vi "PSA Alignment Progress Bar.vi"(8 "error in (no error)":errorcluster, 10 "Time Target (s)":dbl=65.0 format="%#_13g", 11 "VISA resource in":refnum<visa-resource-name>) -> (0 "error out":errorcluster, 2 "Complete?":bool, 3 "VISA resource out":refnum<visa-resource-name>)   [LabVIEW 2014]
panel:
  out "Elapsed Time to Alignment Completion":u32(slide) scale=0.0..60.0
  out "Elapsed Time (s)":u32 format="%<%H:%M:%S>t"
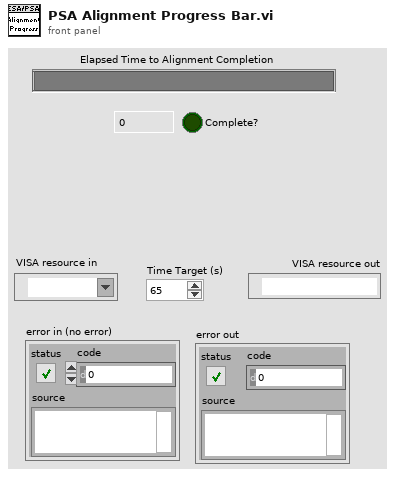
[diagram p1: front panel]
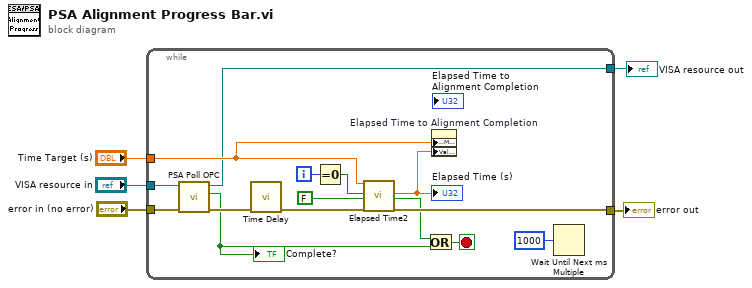
[diagram p0: block diagram]
diagram:
  n1 = while {
    tunnel: [w19] -> w2
    tunnel: "error in (no error)" -> [w12]
    tunnel: "VISA resource in" -> [w10]
    tunnel: "Time Target (s)" -> [w13]
    tunnel: [w6] -> w1
    i -> [w16]
    stop <- w17 stop-if-true
    n2 = call "PSA Poll OPC.vi"("error in (no error)"=w12, "VISA resource name"=w10) -> ("error out"=w11:errorcluster, "OPC Complete?"=w9:bool, "VISA resource name out"=w6:refnum<visa-resource-name>)  [unwired: 7 in]
    "Complete?" <- w9
    n3 = call "Time Delay"("error in (no error)"=w11) -> ("error out"=w20:errorcluster)  [unwired: 10 in]
    n4 = Equal To 0?(x=w16) -> (x = 0?=w15:bool)
    n5 = call "Elapsed Time2"("Time Target (s)"=w13, "Reset"=w15, "Auto Reset"=FALSE, "error in (no error)"=w20) -> ("Elapsed Time (s)"=w8:dbl, "Time has Elapsed"=w18:bool, "error out"=w19:errorcluster)  [unwired: 8 in, 5 out]
    "Elapsed Time (s)" <- w8
    n6 = Or(x=w18, y=w9) -> (x .or. y?=w17:bool)
    n7 = property on="Elapsed Time to Alignment Completion" class="Slide (strict)"("Scale.Maximum"=w13, "Value"=w8) -> ()  [unwired: 2 in, 2 out]
    n8 = Wait Until Next ms Multiple(millisecond multiple=u32 1000) -> ()  [unwired: 1 out]
  }
  "error out" <- w2
  "VISA resource out" <- w1
